vi "输入数据解析.vi"(0 "单个参数补充":dbl, 1 "从板号":dbl=1.0, 2 "主板二维码":string="BNET01", 3 "从板二维码":string="BNET01", 5 "主板引用":refnum<vi>, 7 "从板引用":refnum<vi>, 9 "主板选项":string="三级故障阀值", 11 "枚举":enum16{"主板", "从板"}(ring), 12 "快换":bool caption="快换写入") -> (4 "输出数组":dbl[][](array[numeric]), 6 "数组长度":dbl[](array[numeric]), 8 "循环次数":i32, 10 "命令":u32, 14 "名称":string[](array[string]), 15 "命令序号":u32[](array[numeric]))   [LabVIEW 2013] (continued)
            n304 = Insert Into Array(array=w672, new element=w674) -> (w673:dbl[])  [unwired: 1 in]
          }
          n305 = Build Array(62.0 ("元素")) -> (w664:dbl[])
          n306 = Insert Into Array(array=w650, index=w648, new element #1=w648, new element #2=w648) -> (w649:dbl[])
          n307 = Build Array(u32 5 ("命令序号")) -> (w662:u32[])
          n308 = Build Array(w649) -> (w657:dbl[][])
          n309 = Build Array("温度个数") -> (w653:string[])
        }
        frame "温度起始值" {
          n310 = Unbundle By Name(w702) -> ("项目信息"=w697:refnum<vi>)
          n311 = property class="Tbl (严格)"(reference=w697) -> ("Value"=w696:string[][])  [unwired: 1 in, 2 out]
          n312 = Index Array(array=w696, index (col)=1 ("禁用的索引 (列)")) -> (element=w698:string[])  [unwired: 1 in]
          n313 = Increment(x=w689) -> (x+1=w691:dbl)
          n314 = Multiply(x=w689, y=3.0) -> (x*y=w687:dbl)
          n315 = Add(x=w687, y=23.0) -> (x+y=w690:dbl)
          n316 = Array Subset(array=w698, index=w690, length=w691) -> (w700:string[])
          n317 = Fract/Exp String To Number(string=w700) -> (number=w685:dbl[])  [unwired: 4 out]
          n318 = for {
            tunnel: w685 -> [w709] mode=indexing
            shift-right: [w704] -> w684
            shift-left: dbl[] [] -> [w703]
            n319 = Quotient & Remainder(x=w709, y=256.0) -> (x-y*floor(x/y)=w706:dbl, floor(x/y)=w707:dbl)
            n320 = Build Array(w707, w706) -> (w705:dbl[])
            n321 = Insert Into Array(array=w703, new element=w705) -> (w704:dbl[])  [unwired: 1 in]
          }
          n322 = Build Array(62.0 ("元素")) -> (w695:dbl[])
          n323 = Build Array(u32 6 ("命令序号")) -> (w693:u32[])
          n324 = Build Array(w684) -> (w683:dbl[][])
          n325 = Build Array("温度起始值") -> (w679:string[])
        }
        frame "SOC" {
          # "SOC"
          n326 = Unbundle By Name(w730) -> ("一级故障 4"=w725:refnum<vi>)
          n327 = property class="Clust (严格)"(reference=w725) -> ("Value"=w724:T3)  [unwired: 1 in, 2 out]
          n328 = Unbundle By Name(w724) -> ("SOC(%)"=w722:dbl)
          n329 = call "输入分辨率计算-EV05.vi"("1字节?"=FALSE, "数值"=w722, "分辨率"=0.1) -> ("低字节"=w719:dbl, "高字节1"=w720:dbl)  [unwired: 2 in, 5 out]
          n330 = Build Array(w720, w719) -> (w731:dbl[])
          n331 = Two Button Dialog(message="输入SOC前请确认实际容量己输入" ("消息"), 1:"取消" ("F按钮名称（“取消”）"), 2:"确定" ("T按钮名称（“确定”）")) -> (T button?=w713:bool)
          n332 = case shown="假" w713 {
            tunnel: [0 1] -> w726
            frame False {
            }
            frame True {
            }
          }
          n333 = Build Array("SOC") -> (w714:string[])
          n334 = Build Array(w731) -> (w718:dbl[][])
          n335 = Build Array(2.0 ("单个参数补充")) -> (w717:dbl[])
          n336 = Build Array(u32 7 ("命令序号")) -> (w716:u32[])
        }
        frame "电池额定实际容量" {
          w747 = 256.0 ("y")
          w756 = 256.0 ("y")
          # "电池额定容量,实际容量"
          n337 = Unbundle By Name(w767) -> ("一级故障 4"=w754:refnum<vi>)
          n338 = property class="Clust (严格)"(reference=w754) -> ("Value"=w753:T3)  [unwired: 1 in, 2 out]
          n339 = Unbundle By Name(w753) -> ("电池额定容量(A)"=w751:dbl, "电池实际容量(A)"=w750:dbl)
          n340 = call "输入分辨率计算-EV05.vi"("1字节?"=TRUE, "数值 2"=w750, "数值"=w751, "分辨率"=0.001) -> ("高字节 2"=w743:dbl, "高字节1"=w749:dbl)  [unwired: 1 in, 5 out]
          n341 = Quotient & Remainder(x=w749, y=w756) -> (x-y*floor(x/y)=w760:dbl, floor(x/y)=w762:dbl)
          n342 = Quotient & Remainder(x=w743, y=w747) -> (x-y*floor(x/y)=w739:dbl, floor(x/y)=w744:dbl)
          n343 = Quotient & Remainder(x=w762, y=w756) -> (x-y*floor(x/y)=w759:dbl, floor(x/y)=w761:dbl)
          n344 = Quotient & Remainder(x=w744, y=w747) -> (x-y*floor(x/y)=w740:dbl, floor(x/y)=w745:dbl)
          n345 = Quotient & Remainder(x=w761, y=w756) -> (x-y*floor(x/y)=w758:dbl, floor(x/y)=w757:dbl)
          n346 = Quotient & Remainder(x=w745, y=w747) -> (x-y*floor(x/y)=w741:dbl, floor(x/y)=w746:dbl)
          n347 = Quotient & Remainder(x=w746, y=w747) -> (x-y*floor(x/y)=w742:dbl)  [unwired: 1 out]
          n348 = Quotient & Remainder(x=w757, y=w756) -> (x-y*floor(x/y)=w755:dbl)  [unwired: 1 out]
          n349 = Build Array(w755, w758, w759, w760, w742, w741, w740, w739) -> (w768:dbl[])
          n350 = Build Array(w768) -> (w738:dbl[][])
          n351 = Build Array(8.0 ("单个参数补充")) -> (w737:dbl[])
          n352 = Build Array(u32 8 ("命令序号")) -> (w736:u32[])
          n353 = Build Array("电池额定实际容量") -> (w734:string[])
        }
        frame "配置文件版本" {
          w780 = 8 ("长度")
          # "配置文件版本"
          n354 = Unbundle By Name(w782) -> ("一级故障 4"=w776:refnum<vi>)
          n355 = property class="Clust (严格)"(reference=w776) -> ("Value"=w775:T3)  [unwired: 1 in, 2 out]
          n356 = Unbundle By Name(w775) -> ("配置文件版本"=w774:string)
          n357 = String To Byte Array(string=w774) -> (unsigned byte array=w777:u8[])
          n358 = Array Subset(array=w777, length=w780) -> (w783:u8[])  [unwired: 1 in]
          n359 = Build Array(w783) -> (w773:u8[][])
          n360 = Build Array(w780) -> (w772:i32[])
          n361 = Build Array(u32 9 ("命令序号")) -> (w771:u32[])
          n362 = Build Array("配置文件版本") -> (w769:string[])
        }
        frame "参数修改记录" {
          n363 = Unbundle By Name(w806) -> ("一级故障 4"=w795:refnum<vi>)
          n364 = property class="Clust (严格)"(reference=w795) -> ("Value"=w794:T3)  [unwired: 1 in, 2 out]
          n365 = Unbundle By Name(w794) -> ("使用者"=w793:dbl)
          n366 = Quotient & Remainder(x=w793, y=256.0) -> (x-y*floor(x/y)=w790:dbl, floor(x/y)=w791:dbl)
          n367 = call "当前时间解析-8.6.vi"("需要秒？(T)"=TRUE) -> ("年"=w801:u8, "月"=w800:u8, "日"=w799:u8, "时"=w798:u8, "分"=w797:u8, "秒"=w796:u8)  [unwired: 13 out]
          n368 = Build Array(w791, w790, w801, w800, w799, w798, w797, w796) -> (w807:dbl[])
          n369 = Build Array(w807) -> (w789:dbl[][])
          n370 = Build Array(8.0 ("单个参数补充")) -> (w788:dbl[])
          n371 = Build Array(u32 10 ("命令序号")) -> (w787:u32[])
          n372 = Build Array("参数修改记录") -> (w784:string[])
        }
        frame "校正时钟" {
          n373 = call "当前时间解析-8.6.vi"("需要秒？(T)"=TRUE) -> ("年"=w819:u8, "月"=w818:u8, "日"=w817:u8, "时"=w816:u8, "分"=w815:u8, "秒"=w814:u8)  [unwired: 13 out]
          n374 = Build Array(w819, w818, w817, w816, w815, w814) -> (w824:u8[])
          n375 = Build Array(w824) -> (w813:u8[][])
          n376 = Build Array(6.0 ("单个参数补充")) -> (w812:dbl[])
          n377 = Build Array(u32 14 ("命令序号")) -> (w811:u32[])
          n378 = Build Array("校正时钟") -> (w808:string[])
        }
        frame "车牌号" {
          w836 = 8 ("长度")
          # "车牌号"
          n379 = Unbundle By Name(w838) -> ("一级故障 4"=w832:refnum<vi>)
          n380 = property class="Clust (严格)"(reference=w832) -> ("Value"=w831:T3)  [unwired: 1 in, 2 out]
          n381 = Unbundle By Name(w831) -> ("车架(牌)号"=w830:string)
          n382 = String To Byte Array(string=w830) -> (unsigned byte array=w833:u8[])
          n383 = Array Subset(array=w833, length=w836) -> (w839:u8[])  [unwired: 1 in]
          n384 = Build Array(w839) -> (w829:u8[][])
          n385 = Build Array(w836) -> (w828:i32[])
          n386 = Build Array("车牌号") -> (w825:string[])
          n387 = Build Array(u32 11 ("命令序号")) -> (w827:u32[])
        }
        frame "SOH" {
          n388 = Unbundle By Name(w856) -> ("一级故障 4"=w851:refnum<vi>)
          n389 = property class="Clust (严格)"(reference=w851) -> ("Value"=w850:T3)  [unwired: 1 in, 2 out]
          n390 = Unbundle By Name(w850) -> ("SOH(%)"=w849:dbl)
          n391 = call "输入分辨率计算-EV05.vi"("1字节?"=FALSE, "数值"=w849, "分辨率"=0.1) -> ("低字节"=w845:dbl, "高字节1"=w846:dbl)  [unwired: 2 in, 5 out]
          n392 = Build Array(w846, w845) -> (w857:dbl[])
          n393 = Build Array(w857) -> (w844:dbl[][])
          n394 = Build Array(2.0 ("单个参数补充")) -> (w843:dbl[])
          n395 = Build Array("SOH") -> (w840:string[])
          n396 = Build Array(u32 12 ("命令序号")) -> (w842:u32[])
        }
        frame "一级故障阀值" {
          n397 = Unbundle By Name(w863) -> ("一级故障"=w864:refnum<vi>)
          n398 = property class="Clust (严格)"(reference=w864) -> ("Value"=w862:T4)  [unwired: 1 in, 2 out]
          n399 = for {
            N: 17 -> [_]
            tunnel: w862 -> [w874]
            shift-right: [w871] -> w868
            shift-left: dbl[] [] -> [w872]
            i -> [w875]
            n400 = case shown="11" w875 {
              tunnel: w874 -> [w877 w884 w891 w898 w905 w911 w919 w927 w935 w943 w951 w959 w967 w975 w985 w992 w996]
              tunnel: [w878 w885 w893 w900 w906 w914 w922 w930 w938 w946 w954 w960 w969 w977 w984 w991 w998] -> w873
              frame 0, Default {
                # "总电压过高"
                n401 = Unbundle By Name(w877) -> ("总电压过高"=w876:dbl)
                n402 = call "输入分辨率计算-EV05.vi"("1字节?"=FALSE, "数值"=w876, "分辨率"=0.1) -> ("低字节"=w880:dbl, "高字节1"=w879:dbl)  [unwired: 2 in, 5 out]
                n403 = Build Array(w879, w880) -> (w878:dbl[])
              }
              frame 1 {
                # "总电压过低"
                n404 = Unbundle By Name(w884) -> ("总电压过低"=w883:dbl)
                n405 = call "输入分辨率计算-EV05.vi"("1字节?"=FALSE, "数值"=w883, "分辨率"=0.1) -> ("低字节"=w887:dbl, "高字节1"=w886:dbl)  [unwired: 2 in, 5 out]
                n406 = Build Array(w886, w887) -> (w885:dbl[])
              }
              frame 2 {
                # "温度过高"
                n407 = Unbundle By Name(w891) -> ("温度过高"=w890:dbl)
                n408 = call "输入分辨率计算-EV05.vi"("1字节?"=TRUE, "数值"=w890, "偏移量"=-40.0, "分辨率"=1.0) -> ("高字节1"=w894:dbl)  [unwired: 1 in, 6 out]
                n409 = Build Array(w894) -> (w893:dbl[])
              }
              frame 3 {
                # "温度过低"
                n410 = Unbundle By Name(w898) -> ("温度过低"=w897:dbl)
                n411 = call "输入分辨率计算-EV05.vi"("1字节?"=TRUE, "数值"=w897, "偏移量"=-40.0, "分辨率"=1.0) -> ("高字节1"=w901:dbl)  [unwired: 1 in, 6 out]
                n412 = Build Array(w901) -> (w900:dbl[])
              }
              frame 4 {
                # "整组温度不均衡"
                n413 = Unbundle By Name(w905) -> ("整组温度不均衡"=w904:dbl)
                n414 = call "输入分辨率计算-EV05.vi"("1字节?"=TRUE, "数值"=w904, "分辨率"=1.0) -> ("高字节1"=w907:dbl)  [unwired: 2 in, 6 out]
                n415 = Build Array(w907) -> (w906:dbl[])
              }
              frame 5 {
                # "单组电压不均衡"
                n416 = Unbundle By Name(w911) -> ("单组电压不均衡"=w910:dbl)
                n417 = call "输入分辨率计算-EV05.vi"("1字节?"=FALSE, "数值"=w910, "偏移量"=0.0, "分辨率"=0.001) -> ("低字节"=w912:dbl, "高字节1"=w915:dbl)  [unwired: 1 in, 5 out]
                n418 = Build Array(w915, w912) -> (w914:dbl[])
              }
              frame 6 {
                # "整组电压不均衡"
                n419 = Unbundle By Name(w919) -> ("整组电压不均衡"=w918:dbl)
                n420 = call "输入分辨率计算-EV05.vi"("1字节?"=FALSE, "数值"=w918, "偏移量"=0.0, "分辨率"=0.001) -> ("低字节"=w920:dbl, "高字节1"=w923:dbl)  [unwired: 1 in, 5 out]
                n421 = Build Array(w923, w920) -> (w922:dbl[])
              }
              frame 7 {
                # "单体电压过高"
                n422 = Unbundle By Name(w927) -> ("单体电压过高"=w926:dbl)
                n423 = call "输入分辨率计算-EV05.vi"("1字节?"=FALSE, "数值"=w926, "偏移量"=0.0, "分辨率"=0.001) -> ("低字节"=w928:dbl, "高字节1"=w931:dbl)  [unwired: 1 in, 5 out]
                n424 = Build Array(w931, w928) -> (w930:dbl[])
              }
              frame 8 {
                # "单体电压过低"
                n425 = Unbundle By Name(w935) -> ("单体电压过低"=w934:dbl)
                n426 = call "输入分辨率计算-EV05.vi"("1字节?"=FALSE, "数值"=w934, "偏移量"=0.0, "分辨率"=0.001) -> ("低字节"=w936:dbl, "高字节1"=w939:dbl)  [unwired: 1 in, 5 out]
                n427 = Build Array(w939, w936) -> (w938:dbl[])
              }
              frame 9 {
                # "充电电流过高"
                n428 = Unbundle By Name(w943) -> ("充电电流过高"=w942:dbl)
                n429 = call "输入分辨率计算-EV05.vi"("1字节?"=FALSE, "数值"=w942, "偏移量"=0.0, "分辨率"=0.1) -> ("低字节"=w944:dbl, "高字节1"=w947:dbl)  [unwired: 1 in, 5 out]
                n430 = Build Array(w947, w944) -> (w946:dbl[])
              }
              frame 10 {
                # "放电电流过高"
                n431 = Unbundle By Name(w951) -> ("放电电流过高"=w950:dbl)
                n432 = call "输入分辨率计算-EV05.vi"("1字节?"=FALSE, "数值"=w950, "偏移量"=0.0, "分辨率"=0.1) -> ("低字节"=w952:dbl, "高字节1"=w955:dbl)  [unwired: 1 in, 5 out]
                n433 = Build Array(w955, w952) -> (w954:dbl[])
              }
              frame 11 {
                # "单组温度不均衡"
                n434 = Unbundle By Name(w959) -> ("单组温度不均衡"=w958:dbl)
                n435 = call "输入分辨率计算-EV05.vi"("1字节?"=TRUE, "数值"=w958, "分辨率"=1.0) -> ("高字节1"=w961:dbl)  [unwired: 2 in, 6 out]
                n436 = Build Array(w961) -> (w960:dbl[])
              }
              frame 12 {
                # "SOC过高"
                n437 = Unbundle By Name(w967) -> ("SOC过高"=w966:dbl)
                n438 = call "输入分辨率计算-EV05.vi"("1字节?"=FALSE, "数值"=w966, "偏移量"=0.0, "分辨率"=0.1) -> ("低字节"=w964:dbl, "高字节1"=w965:dbl)  [unwired: 1 in, 5 out]
                n439 = Build Array(w965, w964) -> (w969:dbl[])
              }
              frame 13 {
                # "SOC过低"
                n440 = Unbundle By Name(w975) -> ("SOC过低"=w974:dbl)
                n441 = call "输入分辨率计算-EV05.vi"("1字节?"=FALSE, "数值"=w974, "偏移量"=0.0, "分辨率"=0.1) -> ("低字节"=w972:dbl, "高字节1"=w973:dbl)  [unwired: 1 in, 5 out]
                n442 = Build Array(w973, w972) -> (w977:dbl[])
              }
              frame 14 {
                # "内阻过大"
                n443 = Unbundle By Name(w985) -> ("内阻过大"=w983:dbl)
                n444 = call "输入分辨率计算-EV05.vi"("1字节?"=TRUE, "数值"=w983, "分辨率"=0.1) -> ("高字节1"=w980:dbl)  [unwired: 2 in, 6 out]
                n445 = Build Array(w980) -> (w984:dbl[])
              }
              frame 15 {
                # "极柱温度过高"
                n446 = Unbundle By Name(w992) -> ("极柱温度过高"=w990:dbl)
                n447 = call "输入分辨率计算-EV05.vi"("1字节?"=TRUE, "数值"=w990, "偏移量"=-40.0, "分辨率"=1.0) -> ("高字节1"=w987:dbl)  [unwired: 1 in, 6 out]
                n448 = Build Array(w987) -> (w991:dbl[])
              }
              frame 16 {
                # "SOH过低"
                n449 = Unbundle By Name(w996) -> ("SOH过低"=w995:dbl)
                n450 = call "输入分辨率计算-EV05.vi"("1字节?"=FALSE, "数值"=w995, "偏移量"=0.0, "分辨率"=0.1) -> ("低字节"=w994:dbl, "高字节1"=w993:dbl)  [unwired: 1 in, 5 out]
                n451 = Build Array(w993, w994) -> (w998:dbl[])
              }
            }
            n452 = Insert Into Array(array=w872, new element=w873) -> (w871:dbl[])  [unwired: 1 in]
          }
          n453 = Build Array(w868) -> (w867:dbl[][])
          n454 = Build Array("一级故障阀值") -> (w858:string[])
        }
        frame "温度过高" {
          n455 = Unbundle By Name(w1006) -> ("一级故障"=w1007:refnum<vi>)
          n456 = property class="Clust (严格)"(reference=w1007) -> ("Value"=w1005:T4)  [unwired: 1 in, 2 out]
          n457 = for {
            N: 17 -> [_]
            tunnel: w1005 -> [w1017]
            shift-right: [w1014] -> w1011
            shift-left: dbl[] [] -> [w1015]
            i -> [w1018]
            n458 = case shown="13" w1018 {
              tunnel: w1017 -> [w1019 w1030 w1041 w1051 w1061 w1071 w1083 w1095 w1107 w1119 w1131 w1143 w1157 w1179 w1191 w1200 w1209]
              tunnel: [w1020 w1031 w1042 w1052 w1062 w1073 w1085 w1097 w1109 w1121 w1133 w1144 w1166 w1182 w1190 w1199 w1211] -> w1016
              frame 0, Default {
                # "总电压过高"
                n459 = disable-structure shown="启用" {
                  disable-tunnel: [w1026 w1029] -> w1022
                  disable-tunnel: [w1025 w1029] -> w1021
                  disable-tunnel: w1019 -> [w1024 _]
                  frame Disabled {
                    n460 = Unbundle By Name(w1024) -> ("总电压过高"=w1023:dbl)
                    n461 = call "输入分辨率计算-EV05.vi"("1字节?"=FALSE, "数值"=w1023, "分辨率"=0.1) -> ("低字节"=w1026:dbl, "高字节1"=w1025:dbl)  [unwired: 2 in, 5 out]
                  }
                  frame Enabled {
                    w1029 = 255 ("高字节1")
                  }
                }
                n462 = Build Array(w1021, w1022) -> (w1020:i32[])
              }
              frame 1 {
                # "总电压过低"
                n463 = disable-structure shown="启用" {
                  disable-tunnel: [w1037 w1040] -> w1033
                  disable-tunnel: [w1036 w1040] -> w1032
                  disable-tunnel: w1030 -> [w1035 _]
                  frame Disabled {
                    n464 = Unbundle By Name(w1035) -> ("总电压过低"=w1034:dbl)
                    n465 = call "输入分辨率计算-EV05.vi"("1字节?"=FALSE, "数值"=w1034, "分辨率"=0.1) -> ("低字节"=w1037:dbl, "高字节1"=w1036:dbl)  [unwired: 2 in, 5 out]
                  }
                  frame Enabled {
                    w1040 = 255 ("高字节1")
                  }
                }
                n466 = Build Array(w1032, w1033) -> (w1031:i32[])
              }
              frame 2 {
                # "温度过高"
                n467 = disable-structure shown="启用" {
                  disable-tunnel: [w1047 255 ("高字节1")] -> w1043
                  disable-tunnel: w1041 -> [w1045 _]
                  frame Enabled {
                    n468 = Unbundle By Name(w1045) -> ("温度过高"=w1044:dbl)
                    n469 = call "输入分辨率计算-EV05.vi"("1字节?"=TRUE, "数值"=w1044, "偏移量"=-40.0, "分辨率"=1.0) -> ("高字节1"=w1047:dbl)  [unwired: 1 in, 6 out]
                  }
                  frame Disabled {
                  }
                }
                n470 = Build Array(w1043) -> (w1042:dbl[])
              }
              frame 3 {
                # "温度过低"
                n471 = disable-structure shown="启用" {
                  disable-tunnel: [w1057 255 ("高字节1")] -> w1053
                  disable-tunnel: w1051 -> [w1055 _]
                  frame Disabled {
                    n472 = Unbundle By Name(w1055) -> ("温度过低"=w1054:dbl)
                    n473 = call "输入分辨率计算-EV05.vi"("1字节?"=TRUE, "数值"=w1054, "偏移量"=-40.0, "分辨率"=1.0) -> ("高字节1"=w1057:dbl)  [unwired: 1 in, 6 out]
                  }
                  frame Enabled {
                  }
                }
                n474 = Build Array(w1053) -> (w1052:i32[])
              }
              frame 4 {
                # "整组温度不均衡"
                n475 = disable-structure shown="启用" {
                  disable-tunnel: [w1067 255 ("高字节1")] -> w1063
                  disable-tunnel: w1061 -> [w1065 _]
                  frame Disabled {
                    n476 = Unbundle By Name(w1065) -> ("整组温度不均衡"=w1064:dbl)
                    n477 = call "输入分辨率计算-EV05.vi"("1字节?"=TRUE, "数值"=w1064, "偏移量"=0.0, "分辨率"=1.0) -> ("高字节1"=w1067:dbl)  [unwired: 1 in, 6 out]
                  }
                  frame Enabled {
                  }
                }
                n478 = Build Array(w1063) -> (w1062:i32[])
              }
              frame 5 {
                # "单组电压不均衡"
                n479 = disable-structure shown="启用" {
                  disable-tunnel: [w1079 w1082] -> w1074
                  disable-tunnel: [w1077 w1082] -> w1072
                  disable-tunnel: w1071 -> [w1076 _]
                  frame Disabled {
                    n480 = Unbundle By Name(w1076) -> ("单组电压不均衡"=w1075:dbl)
                    n481 = call "输入分辨率计算-EV05.vi"("1字节?"=FALSE, "数值"=w1075, "偏移量"=0.0, "分辨率"=0.001) -> ("低字节"=w1077:dbl, "高字节1"=w1079:dbl)  [unwired: 1 in, 5 out]
                  }
                  frame Enabled {
                    w1082 = 255 ("高字节1")
                  }
                }
                n482 = Build Array(w1074, w1072) -> (w1073:i32[])
              }
              frame 6 {
                # "整组电压不均衡"
                n483 = disable-structure shown="启用" {
                  disable-tunnel: [w1091 w1094] -> w1086
                  disable-tunnel: [w1089 w1094] -> w1084
                  disable-tunnel: w1083 -> [w1088 _]
                  frame Disabled {
                    n484 = Unbundle By Name(w1088) -> ("整组电压不均衡"=w1087:dbl)
                    n485 = call "输入分辨率计算-EV05.vi"("1字节?"=FALSE, "数值"=w1087, "偏移量"=0.0, "分辨率"=0.001) -> ("低字节"=w1089:dbl, "高字节1"=w1091:dbl)  [unwired: 1 in, 5 out]
                  }
                  frame Enabled {
                    w1094 = 255 ("高字节1")
                  }
                }
                n486 = Build Array(w1086, w1084) -> (w1085:i32[])
              }
              frame 7 {
                # "单体电压过高"
                n487 = disable-structure shown="启用" {
                  disable-tunnel: [w1103 w1106] -> w1098
                  disable-tunnel: [w1101 w1106] -> w1096
                  disable-tunnel: w1095 -> [w1100 _]
                  frame Disabled {
                    n488 = Unbundle By Name(w1100) -> ("单体电压过高"=w1099:dbl)
                    n489 = call "输入分辨率计算-EV05.vi"("1字节?"=FALSE, "数值"=w1099, "偏移量"=0.0, "分辨率"=0.001) -> ("低字节"=w1101:dbl, "高字节1"=w1103:dbl)  [unwired: 1 in, 5 out]
                  }
                  frame Enabled {
                    w1106 = 255 ("高字节1")
                  }
                }
                n490 = Build Array(w1098, w1096) -> (w1097:i32[])
              }
              frame 8 {
                # "单体电压过低"
                n491 = disable-structure shown="启用" {
                  disable-tunnel: [w1115 w1118] -> w1110
                  disable-tunnel: [w1113 w1118] -> w1108
                  disable-tunnel: w1107 -> [w1112 _]
                  frame Disabled {
                    n492 = Unbundle By Name(w1112) -> ("单体电压过低"=w1111:dbl)
                    n493 = call "输入分辨率计算-EV05.vi"("1字节?"=FALSE, "数值"=w1111, "偏移量"=0.0, "分辨率"=0.001) -> ("低字节"=w1113:dbl, "高字节1"=w1115:dbl)  [unwired: 1 in, 5 out]
                  }
                  frame Enabled {
                    w1118 = 255 ("高字节1")
                  }
                }
                n494 = Build Array(w1110, w1108) -> (w1109:i32[])
              }
              frame 9 {
                # "充电电流过高"
                n495 = disable-structure shown="启用" {
                  disable-tunnel: [w1127 w1130] -> w1122
                  disable-tunnel: [w1125 w1130] -> w1120
                  disable-tunnel: w1119 -> [w1124 _]
                  frame Disabled {
                    n496 = Unbundle By Name(w1124) -> ("充电电流过高"=w1123:dbl)
                    n497 = call "输入分辨率计算-EV05.vi"("1字节?"=FALSE, "数值"=w1123, "偏移量"=-3000.0, "分辨率"=0.1) -> ("低字节"=w1125:dbl, "高字节1"=w1127:dbl)  [unwired: 1 in, 5 out]
                  }
                  frame Enabled {
                    w1130 = 255 ("高字节1")
                  }
                }
                n498 = Build Array(w1122, w1120) -> (w1121:i32[])
              }
              frame 10 {
                # "放电电流过高"
                n499 = disable-structure shown="启用" {
                  disable-tunnel: [w1139 w1142] -> w1134
                  disable-tunnel: [w1137 w1142] -> w1132
                  disable-tunnel: w1131 -> [w1136 _]
                  frame Disabled {
                    n500 = Unbundle By Name(w1136) -> ("放电电流过高"=w1135:dbl)
                    n501 = call "输入分辨率计算-EV05.vi"("1字节?"=FALSE, "数值"=w1135, "偏移量"=-3000.0, "分辨率"=0.1) -> ("低字节"=w1137:dbl, "高字节1"=w1139:dbl)  [unwired: 1 in, 5 out]
                  }
                  frame Enabled {
                    w1142 = 255 ("高字节1")
                  }
                }
                n502 = Build Array(w1134, w1132) -> (w1133:i32[])
              }
              frame 11 {
                # "单组温度不均衡"
                n503 = disable-structure shown="启用" {
                  disable-tunnel: [w1149 255 ("高字节1")] -> w1145
                  disable-tunnel: w1143 -> [w1147 _]
                  frame Disabled {
                    n504 = Unbundle By Name(w1147) -> ("单组温度不均衡"=w1146:dbl)
                    n505 = call "输入分辨率计算-EV05.vi"("1字节?"=TRUE, "数值"=w1146, "偏移量"=0.0, "分辨率"=1.0) -> ("高字节1"=w1149:dbl)  [unwired: 1 in, 6 out]
                  }
                  frame Enabled {
                  }
                }
                n506 = Build Array(w1145) -> (w1144:i32[])
              }
              frame 12 {
                # "SOC过高"
                n507 = Unbundle By Name(w1157) -> ("SOC过高"=w1156:dbl)
                n508 = call "输入分辨率计算-EV05.vi"("1字节?"=FALSE, "数值"=w1156, "偏移量"=0.0, "分辨率"=0.1) -> ("低字节"=w1158:dbl, "高字节1"=w1159:dbl)  [unwired: 1 in, 5 out]
                n509 = call "二进制解析-8.6.vi"("索引"=4, "数值"=w1159) -> ("低位子数组"=w1162:i32[])  [unwired: 3 out]
                n510 = call "二进制解析-8.6.vi"("索引"=4, "数值"=w1158) -> ("低位子数组"=w1154:i32[], "高位子数组"=w1161:i32[])  [unwired: 2 out]
                n511 = Insert Into Array(array=w1162, new element=w1161) -> (w1160:i32[])  [unwired: 1 in]
                n512 = call "数值二进制转十进制-8.6.vi"("子数组"=w1160) -> ("十进制数值"=w1155:i32)  [unwired: 4 out]
                n513 = disable-structure shown="启用" {
                  disable-tunnel: w1155 -> [w1170 _]
                  disable-tunnel: [w1170 255 ("高字节1")] -> w1153
                  disable-tunnel: [w1169 i32[] [] ("低位子数组 20")] -> _
                  disable-tunnel: w1154 -> [w1169 _]
                  frame Disabled {
                  }
                  frame Enabled {
                  }
                }
                n514 = Build Array(w1153, w1153) -> (w1166:i32[])
              }
              frame 13 {
                # "SOC过低"
                n515 = Unbundle By Name(w1179) -> ("SOC过低"=w1178:dbl)
                n516 = call "输入分辨率计算-EV05.vi"("1字节?"=FALSE, "数值"=w1178, "偏移量"=0.0, "分辨率"=0.1) -> ("低字节"=w1176:dbl, "高字节1"=w1177:dbl)  [unwired: 1 in, 5 out]
                n517 = call "二进制解析-8.6.vi"("索引"=4, "数值"=w1177) -> ("低位子数组"=w1174:i32[])  [unwired: 3 out]
                n518 = disable-structure shown="启用" {
                  disable-tunnel: w1176 -> [w1186 _]
                  disable-tunnel: [w1186 255 ("高字节1")] -> w1175
                  disable-tunnel: w1174 -> [w1185 _]
                  disable-tunnel: [_ 255 ("高字节1")] -> w1173
                  frame Disabled {
                    (unwired) i32[] [] ("低位子数组 4")
                  }
                  frame Enabled {
                  }
                }
                n519 = Build Array(w1173, w1175) -> (w1182:i32[])
              }
              frame 14 {
                # "内阻过大"
                n520 = disable-structure shown="启用" {
                  disable-tunnel: w1191 -> [w1196 _]
                  disable-tunnel: [w1192 255 ("高字节1")] -> w1189
                  frame Disabled {
                    n521 = Unbundle By Name(w1196) -> ("内阻过大"=w1195:dbl)
                    n522 = call "输入分辨率计算-EV05.vi"("1字节?"=TRUE, "数值"=w1195, "分辨率"=0.1) -> ("高字节1"=w1192:dbl)  [unwired: 2 in, 6 out]
                  }
                  frame Enabled {
                  }
                }
                n523 = Build Array(w1189) -> (w1190:i32[])
              }
              frame 15 {
                # "极柱温度过高"
                n524 = disable-structure shown="启用" {
                  disable-tunnel: w1200 -> [w1206 _]
                  disable-tunnel: [w1202 255 ("高字节1")] -> w1198
                  frame Disabled {
                    n525 = Unbundle By Name(w1206) -> ("极柱温度过高"=w1205:dbl)
                    n526 = call "输入分辨率计算-EV05.vi"("1字节?"=TRUE, "数值"=w1205, "偏移量"=-40.0, "分辨率"=1.0) -> ("高字节1"=w1202:dbl)  [unwired: 1 in, 6 out]
                  }
                  frame Enabled {
                  }
                }
                n527 = Build Array(w1198) -> (w1199:i32[])
              }
              frame 16 {
                # "SOH过低"
                n528 = disable-structure shown="启用" {
                  disable-tunnel: [w1223 w1231] -> w1210
                  disable-tunnel: w1209 -> [w1220 _]
                  disable-tunnel: [w1212 w1231] -> w1208
                  frame Disabled {
                    n529 = Unbundle By Name(w1220) -> ("SOH过低"=w1219:dbl)
                    n530 = call "输入分辨率计算-EV05.vi"("1字节?"=FALSE, "数值"=w1219, "偏移量"=0.0, "分辨率"=0.1) -> ("低字节"=w1221:dbl, "高字节1"=w1222:dbl)  [unwired: 1 in, 5 out]
                    n531 = call "二进制解析-8.6.vi"("索引"=4, "数值"=w1222) -> ("低位子数组"=w1225:i32[])  [unwired: 3 out]
                    n532 = call "二进制解析-8.6.vi"("索引"=4, "数值"=w1221) -> ("低位子数组"=w1214:i32[], "高位子数组"=w1224:i32[])  [unwired: 2 out]
                    n533 = call "二进制解析-8.6.vi"("索引"=4, "数值"=0) -> ("低位子数组"=w1215:i32[])  [unwired: 3 out]
                    n534 = Insert Into Array(array=w1225, new element=w1224) -> (w1218:i32[])  [unwired: 1 in]
                    n535 = Insert Into Array(array=w1214, new element=w1215) -> (w1213:i32[])  [unwired: 1 in]
                    n536 = call "数值二进制转十进制-8.6.vi"("子数组"=w1218) -> ("十进制数值"=w1223:i32)  [unwired: 4 out]
                    n537 = call "数值二进制转十进制-8.6.vi"("子数组"=w1213) -> ("十进制数值"=w1212:i32)  [unwired: 4 out]
                  }
                  frame Enabled {
                    w1231 = 255 ("高字节1")
                  }
                }
                n538 = Build Array(w1210, w1208) -> (w1211:i32[])
              }
            }
            n539 = Insert Into Array(array=w1015, new element=w1016) -> (w1014:dbl[])  [unwired: 1 in]
          }
          n540 = Build Array(w1011) -> (w1010:dbl[][])
          n541 = Build Array("一级故障阀值") -> (w1001:string[])
        }
        frame "总电压过高" {
          n542 = Unbundle By Name(w1237) -> ("一级故障"=w1238:refnum<vi>)
          n543 = property class="Clust (严格)"(reference=w1238) -> ("Value"=w1236:T4)  [unwired: 1 in, 2 out]
          n544 = for {
            N: 17 -> [_]
            tunnel: w1236 -> [w1248]
            shift-right: [w1245] -> w1242
            shift-left: dbl[] [] -> [w1246]
            i -> [w1249]
            n545 = case shown="13" w1249 {
              tunnel: w1248 -> [w1250 w1261 w1272 w1282 w1292 w1302 w1314 w1326 w1338 w1350 w1362 w1374 w1388 w1410 w1422 w1431 w1440]
              tunnel: [w1251 w1262 w1273 w1283 w1293 w1304 w1316 w1328 w1340 w1352 w1364 w1375 w1397 w1413 w1421 w1430 w1442] -> w1247
              frame 0, Default {
                # "总电压过高"
                n546 = disable-structure shown="启用" {
                  disable-tunnel: [w1257 w1260] -> w1253
                  disable-tunnel: [w1256 w1260] -> w1252
                  disable-tunnel: w1250 -> [w1255 _]
                  frame Enabled {
                    n547 = Unbundle By Name(w1255) -> ("总电压过高"=w1254:dbl)
                    n548 = call "输入分辨率计算-EV05.vi"("1字节?"=FALSE, "数值"=w1254, "分辨率"=0.1) -> ("低字节"=w1257:dbl, "高字节1"=w1256:dbl)  [unwired: 2 in, 5 out]
                  }
                  frame Disabled {
                    w1260 = 255 ("高字节1")
                  }
                }
                n549 = Build Array(w1252, w1253) -> (w1251:dbl[])
              }
              frame 1 {
                # "总电压过低"
                n550 = disable-structure shown="启用" {
                  disable-tunnel: [w1268 w1271] -> w1264
                  disable-tunnel: [w1267 w1271] -> w1263
                  disable-tunnel: w1261 -> [w1266 _]
                  frame Disabled {
                    n551 = Unbundle By Name(w1266) -> ("总电压过低"=w1265:dbl)
                    n552 = call "输入分辨率计算-EV05.vi"("1字节?"=FALSE, "数值"=w1265, "分辨率"=0.1) -> ("低字节"=w1268:dbl, "高字节1"=w1267:dbl)  [unwired: 2 in, 5 out]
                  }
                  frame Enabled {
                    w1271 = 255 ("高字节1")
                  }
                }
                n553 = Build Array(w1263, w1264) -> (w1262:i32[])
              }
              frame 2 {
                # "温度过高"
                n554 = disable-structure shown="启用" {
                  disable-tunnel: [w1278 255 ("高字节1")] -> w1274
                  disable-tunnel: w1272 -> [w1276 _]
                  frame Disabled {
                    n555 = Unbundle By Name(w1276) -> ("温度过高"=w1275:dbl)
                    n556 = call "输入分辨率计算-EV05.vi"("1字节?"=TRUE, "数值"=w1275, "偏移量"=-40.0, "分辨率"=1.0) -> ("高字节1"=w1278:dbl)  [unwired: 1 in, 6 out]
                  }
                  frame Enabled {
                  }
                }
                n557 = Build Array(w1274) -> (w1273:i32[])
              }
              frame 3 {
                # "温度过低"
                n558 = disable-structure shown="启用" {
                  disable-tunnel: [w1288 255 ("高字节1")] -> w1284
                  disable-tunnel: w1282 -> [w1286 _]
                  frame Disabled {
                    n559 = Unbundle By Name(w1286) -> ("温度过低"=w1285:dbl)
                    n560 = call "输入分辨率计算-EV05.vi"("1字节?"=TRUE, "数值"=w1285, "偏移量"=-40.0, "分辨率"=1.0) -> ("高字节1"=w1288:dbl)  [unwired: 1 in, 6 out]
                  }
                  frame Enabled {
                  }
                }
                n561 = Build Array(w1284) -> (w1283:i32[])
              }
              frame 4 {
                # "整组温度不均衡"
                n562 = disable-structure shown="启用" {
                  disable-tunnel: [w1298 255 ("高字节1")] -> w1294
                  disable-tunnel: w1292 -> [w1296 _]
                  frame Disabled {
                    n563 = Unbundle By Name(w1296) -> ("整组温度不均衡"=w1295:dbl)
                    n564 = call "输入分辨率计算-EV05.vi"("1字节?"=TRUE, "数值"=w1295, "偏移量"=0.0, "分辨率"=1.0) -> ("高字节1"=w1298:dbl)  [unwired: 1 in, 6 out]
                  }
                  frame Enabled {
                  }
                }
                n565 = Build Array(w1294) -> (w1293:i32[])
              }
              frame 5 {
                # "单组电压不均衡"
                n566 = disable-structure shown="启用" {
                  disable-tunnel: [w1310 w1313] -> w1305
                  disable-tunnel: [w1308 w1313] -> w1303
                  disable-tunnel: w1302 -> [w1307 _]
                  frame Disabled {
                    n567 = Unbundle By Name(w1307) -> ("单组电压不均衡"=w1306:dbl)
                    n568 = call "输入分辨率计算-EV05.vi"("1字节?"=FALSE, "数值"=w1306, "偏移量"=0.0, "分辨率"=0.001) -> ("低字节"=w1308:dbl, "高字节1"=w1310:dbl)  [unwired: 1 in, 5 out]
                  }
                  frame Enabled {
                    w1313 = 255 ("高字节1")
                  }
                }
                n569 = Build Array(w1305, w1303) -> (w1304:i32[])
              }
              frame 6 {
                # "整组电压不均衡"
                n570 = disable-structure shown="启用" {
                  disable-tunnel: [w1322 w1325] -> w1317
                  disable-tunnel: [w1320 w1325] -> w1315
                  disable-tunnel: w1314 -> [w1319 _]
                  frame Disabled {
                    n571 = Unbundle By Name(w1319) -> ("整组电压不均衡"=w1318:dbl)
                    n572 = call "输入分辨率计算-EV05.vi"("1字节?"=FALSE, "数值"=w1318, "偏移量"=0.0, "分辨率"=0.001) -> ("低字节"=w1320:dbl, "高字节1"=w1322:dbl)  [unwired: 1 in, 5 out]
                  }
                  frame Enabled {
                    w1325 = 255 ("高字节1")
                  }
                }
                n573 = Build Array(w1317, w1315) -> (w1316:i32[])
              }
              frame 7 {
                # "单体电压过高"
                n574 = disable-structure shown="启用" {
                  disable-tunnel: [w1334 w1337] -> w1329
                  disable-tunnel: [w1332 w1337] -> w1327
                  disable-tunnel: w1326 -> [w1331 _]
                  frame Disabled {
                    n575 = Unbundle By Name(w1331) -> ("单体电压过高"=w1330:dbl)
                    n576 = call "输入分辨率计算-EV05.vi"("1字节?"=FALSE, "数值"=w1330, "偏移量"=0.0, "分辨率"=0.001) -> ("低字节"=w1332:dbl, "高字节1"=w1334:dbl)  [unwired: 1 in, 5 out]
                  }
                  frame Enabled {
                    w1337 = 255 ("高字节1")
                  }
                }
                n577 = Build Array(w1329, w1327) -> (w1328:i32[])
              }
              frame 8 {
                # "单体电压过低"
                n578 = disable-structure shown="启用" {
                  disable-tunnel: [w1346 w1349] -> w1341
                  disable-tunnel: [w1344 w1349] -> w1339
                  disable-tunnel: w1338 -> [w1343 _]
                  frame Disabled {
                    n579 = Unbundle By Name(w1343) -> ("单体电压过低"=w1342:dbl)
                    n580 = call "输入分辨率计算-EV05.vi"("1字节?"=FALSE, "数值"=w1342, "偏移量"=0.0, "分辨率"=0.001) -> ("低字节"=w1344:dbl, "高字节1"=w1346:dbl)  [unwired: 1 in, 5 out]
                  }
                  frame Enabled {
                    w1349 = 255 ("高字节1")
                  }
                }
                n581 = Build Array(w1341, w1339) -> (w1340:i32[])
              }
              frame 9 {
                # "充电电流过高"
                n582 = disable-structure shown="启用" {
                  disable-tunnel: [w1358 w1361] -> w1353
                  disable-tunnel: [w1356 w1361] -> w1351
                  disable-tunnel: w1350 -> [w1355 _]
                  frame Disabled {
                    n583 = Unbundle By Name(w1355) -> ("充电电流过高"=w1354:dbl)
                    n584 = call "输入分辨率计算-EV05.vi"("1字节?"=FALSE, "数值"=w1354, "偏移量"=-3000.0, "分辨率"=0.1) -> ("低字节"=w1356:dbl, "高字节1"=w1358:dbl)  [unwired: 1 in, 5 out]
                  }
                  frame Enabled {
                    w1361 = 255 ("高字节1")
                  }
                }
                n585 = Build Array(w1353, w1351) -> (w1352:i32[])
              }
              frame 10 {
                # "放电电流过高"
                n586 = disable-structure shown="启用" {
                  disable-tunnel: [w1370 w1373] -> w1365
                  disable-tunnel: [w1368 w1373] -> w1363
                  disable-tunnel: w1362 -> [w1367 _]
                  frame Disabled {
                    n587 = Unbundle By Name(w1367) -> ("放电电流过高"=w1366:dbl)
                    n588 = call "输入分辨率计算-EV05.vi"("1字节?"=FALSE, "数值"=w1366, "偏移量"=-3000.0, "分辨率"=0.1) -> ("低字节"=w1368:dbl, "高字节1"=w1370:dbl)  [unwired: 1 in, 5 out]
                  }
                  frame Enabled {
                    w1373 = 255 ("高字节1")
                  }
                }
                n589 = Build Array(w1365, w1363) -> (w1364:i32[])
              }
              frame 11 {
                # "单组温度不均衡"
                n590 = disable-structure shown="启用" {
                  disable-tunnel: [w1380 255 ("高字节1")] -> w1376
                  disable-tunnel: w1374 -> [w1378 _]
                  frame Disabled {
                    n591 = Unbundle By Name(w1378) -> ("单组温度不均衡"=w1377:dbl)
                    n592 = call "输入分辨率计算-EV05.vi"("1字节?"=TRUE, "数值"=w1377, "偏移量"=0.0, "分辨率"=1.0) -> ("高字节1"=w1380:dbl)  [unwired: 1 in, 6 out]
                  }
                  frame Enabled {
                  }
                }
                n593 = Build Array(w1376) -> (w1375:i32[])
              }
              frame 12 {
                # "SOC过高"
                n594 = Unbundle By Name(w1388) -> ("SOC过高"=w1387:dbl)
                n595 = call "输入分辨率计算-EV05.vi"("1字节?"=FALSE, "数值"=w1387, "偏移量"=0.0, "分辨率"=0.1) -> ("低字节"=w1389:dbl, "高字节1"=w1390:dbl)  [unwired: 1 in, 5 out]
                n596 = call "二进制解析-8.6.vi"("索引"=4, "数值"=w1390) -> ("低位子数组"=w1393:i32[])  [unwired: 3 out]
                n597 = call "二进制解析-8.6.vi"("索引"=4, "数值"=w1389) -> ("低位子数组"=w1385:i32[], "高位子数组"=w1392:i32[])  [unwired: 2 out]
                n598 = Insert Into Array(array=w1393, new element=w1392) -> (w1391:i32[])  [unwired: 1 in]
                n599 = call "数值二进制转十进制-8.6.vi"("子数组"=w1391) -> ("十进制数值"=w1386:i32)  [unwired: 4 out]
                n600 = disable-structure shown="启用" {
                  disable-tunnel: w1386 -> [w1401 _]
                  disable-tunnel: [w1401 255 ("高字节1")] -> w1384
                  disable-tunnel: [w1400 i32[] [] ("低位子数组 20")] -> _
                  disable-tunnel: w1385 -> [w1400 _]
                  frame Disabled {
                  }
                  frame Enabled {
                  }
                }
                n601 = Build Array(w1384, w1384) -> (w1397:i32[])
              }
              frame 13 {
                # "SOC过低"
                n602 = Unbundle By Name(w1410) -> ("SOC过低"=w1409:dbl)
                n603 = call "输入分辨率计算-EV05.vi"("1字节?"=FALSE, "数值"=w1409, "偏移量"=0.0, "分辨率"=0.1) -> ("低字节"=w1407:dbl, "高字节1"=w1408:dbl)  [unwired: 1 in, 5 out]
                n604 = call "二进制解析-8.6.vi"("索引"=4, "数值"=w1408) -> ("低位子数组"=w1405:i32[])  [unwired: 3 out]
                n605 = disable-structure shown="启用" {
                  disable-tunnel: w1407 -> [w1417 _]
                  disable-tunnel: [w1417 255 ("高字节1")] -> w1406
                  disable-tunnel: w1405 -> [w1416 _]
                  disable-tunnel: [_ 255 ("高字节1")] -> w1404
                  frame Disabled {
                    (unwired) i32[] [] ("低位子数组 4")
                  }
                  frame Enabled {
                  }
                }
                n606 = Build Array(w1404, w1406) -> (w1413:i32[])
              }
              frame 14 {
                # "内阻过大"
                n607 = disable-structure shown="启用" {
                  disable-tunnel: w1422 -> [w1427 _]
                  disable-tunnel: [w1423 255 ("高字节1")] -> w1420
                  frame Disabled {
                    n608 = Unbundle By Name(w1427) -> ("内阻过大"=w1426:dbl)
                    n609 = call "输入分辨率计算-EV05.vi"("1字节?"=TRUE, "数值"=w1426, "分辨率"=0.1) -> ("高字节1"=w1423:dbl)  [unwired: 2 in, 6 out]
                  }
                  frame Enabled {
                  }
                }
                n610 = Build Array(w1420) -> (w1421:i32[])
              }
              frame 15 {
                # "极柱温度过高"
                n611 = disable-structure shown="启用" {
                  disable-tunnel: w1431 -> [w1437 _]
                  disable-tunnel: [w1433 255 ("高字节1")] -> w1429
                  frame Disabled {
                    n612 = Unbundle By Name(w1437) -> ("极柱温度过高"=w1436:dbl)
                    n613 = call "输入分辨率计算-EV05.vi"("1字节?"=TRUE, "数值"=w1436, "偏移量"=-40.0, "分辨率"=1.0) -> ("高字节1"=w1433:dbl)  [unwired: 1 in, 6 out]
                  }
                  frame Enabled {
                  }
                }
                n614 = Build Array(w1429) -> (w1430:i32[])
              }
              frame 16 {
                # "SOH过低"
                n615 = disable-structure shown="启用" {
                  disable-tunnel: [w1454 w1462] -> w1441
                  disable-tunnel: w1440 -> [w1451 _]
                  disable-tunnel: [w1443 w1462] -> w1439
                  frame Disabled {
                    n616 = Unbundle By Name(w1451) -> ("SOH过低"=w1450:dbl)
                    n617 = call "输入分辨率计算-EV05.vi"("1字节?"=FALSE, "数值"=w1450, "偏移量"=0.0, "分辨率"=0.1) -> ("低字节"=w1452:dbl, "高字节1"=w1453:dbl)  [unwired: 1 in, 5 out]
                    n618 = call "二进制解析-8.6.vi"("索引"=4, "数值"=w1453) -> ("低位子数组"=w1456:i32[])  [unwired: 3 out]
                    n619 = call "二进制解析-8.6.vi"("索引"=4, "数值"=w1452) -> ("低位子数组"=w1445:i32[], "高位子数组"=w1455:i32[])  [unwired: 2 out]
                    n620 = call "二进制解析-8.6.vi"("索引"=4, "数值"=0) -> ("低位子数组"=w1446:i32[])  [unwired: 3 out]
                    n621 = Insert Into Array(array=w1456, new element=w1455) -> (w1449:i32[])  [unwired: 1 in]
                    n622 = Insert Into Array(array=w1445, new element=w1446) -> (w1444:i32[])  [unwired: 1 in]
                    n623 = call "数值二进制转十进制-8.6.vi"("子数组"=w1449) -> ("十进制数值"=w1454:i32)  [unwired: 4 out]
                    n624 = call "数值二进制转十进制-8.6.vi"("子数组"=w1444) -> ("十进制数值"=w1443:i32)  [unwired: 4 out]
                  }
                  frame Enabled {
                    w1462 = 255 ("高字节1")
                  }
                }
                n625 = Build Array(w1441, w1439) -> (w1442:i32[])
              }
            }
            n626 = Insert Into Array(array=w1246, new element=w1247) -> (w1245:dbl[])  [unwired: 1 in]
          }
          n627 = Build Array(w1242) -> (w1241:dbl[][])
          n628 = Build Array("一级故障阀值") -> (w1232:string[])
        }
        frame "总电压过低" {
          n629 = Unbundle By Name(w1468) -> ("一级故障"=w1469:refnum<vi>)
          n630 = property class="Clust (严格)"(reference=w1469) -> ("Value"=w1467:T4)  [unwired: 1 in, 2 out]
          n631 = for {
            N: 17 -> [_]
            tunnel: w1467 -> [w1479]
            shift-right: [w1476] -> w1473
            shift-left: dbl[] [] -> [w1477]
            i -> [w1480]
            n632 = case shown="13" w1480 {
              tunnel: w1479 -> [w1481 w1492 w1503 w1513 w1523 w1533 w1545 w1557 w1569 w1581 w1593 w1605 w1619 w1641 w1653 w1662 w1671]
              tunnel: [w1482 w1493 w1504 w1514 w1524 w1535 w1547 w1559 w1571 w1583 w1595 w1606 w1628 w1644 w1652 w1661 w1673] -> w1478
              frame 0, Default {
                # "总电压过高"
                n633 = disable-structure shown="启用" {
                  disable-tunnel: [w1488 w1491] -> w1484
                  disable-tunnel: [w1487 w1491] -> w1483
                  disable-tunnel: w1481 -> [w1486 _]
                  frame Disabled {
                    n634 = Unbundle By Name(w1486) -> ("总电压过高"=w1485:dbl)
                    n635 = call "输入分辨率计算-EV05.vi"("1字节?"=FALSE, "数值"=w1485, "分辨率"=0.1) -> ("低字节"=w1488:dbl, "高字节1"=w1487:dbl)  [unwired: 2 in, 5 out]
                  }
                  frame Enabled {
                    w1491 = 255 ("高字节1")
                  }
                }
                n636 = Build Array(w1483, w1484) -> (w1482:i32[])
              }
              frame 1 {
                # "总电压过低"
                n637 = disable-structure shown="启用" {
                  disable-tunnel: [w1499 w1502] -> w1495
                  disable-tunnel: [w1498 w1502] -> w1494
                  disable-tunnel: w1492 -> [w1497 _]
                  frame Enabled {
                    n638 = Unbundle By Name(w1497) -> ("总电压过低"=w1496:dbl)
                    n639 = call "输入分辨率计算-EV05.vi"("1字节?"=FALSE, "数值"=w1496, "分辨率"=0.1) -> ("低字节"=w1499:dbl, "高字节1"=w1498:dbl)  [unwired: 2 in, 5 out]
                  }
                  frame Disabled {
                    w1502 = 255 ("高字节1")
                  }
                }
                n640 = Build Array(w1494, w1495) -> (w1493:dbl[])
              }
              frame 2 {
                # "温度过高"
                n641 = disable-structure shown="启用" {
                  disable-tunnel: [w1509 255 ("高字节1")] -> w1505
                  disable-tunnel: w1503 -> [w1507 _]
                  frame Disabled {
                    n642 = Unbundle By Name(w1507) -> ("温度过高"=w1506:dbl)
                    n643 = call "输入分辨率计算-EV05.vi"("1字节?"=TRUE, "数值"=w1506, "偏移量"=-40.0, "分辨率"=1.0) -> ("高字节1"=w1509:dbl)  [unwired: 1 in, 6 out]
                  }
                  frame Enabled {
                  }
                }
                n644 = Build Array(w1505) -> (w1504:i32[])
              }
              frame 3 {
                # "温度过低"
                n645 = disable-structure shown="启用" {
                  disable-tunnel: [w1519 255 ("高字节1")] -> w1515
                  disable-tunnel: w1513 -> [w1517 _]
                  frame Disabled {
                    n646 = Unbundle By Name(w1517) -> ("温度过低"=w1516:dbl)
                    n647 = call "输入分辨率计算-EV05.vi"("1字节?"=TRUE, "数值"=w1516, "偏移量"=-40.0, "分辨率"=1.0) -> ("高字节1"=w1519:dbl)  [unwired: 1 in, 6 out]
                  }
                  frame Enabled {
                  }
                }
                n648 = Build Array(w1515) -> (w1514:i32[])
              }
              frame 4 {
                # "整组温度不均衡"
                n649 = disable-structure shown="启用" {
                  disable-tunnel: [w1529 255 ("高字节1")] -> w1525
                  disable-tunnel: w1523 -> [w1527 _]
                  frame Disabled {
                    n650 = Unbundle By Name(w1527) -> ("整组温度不均衡"=w1526:dbl)
                    n651 = call "输入分辨率计算-EV05.vi"("1字节?"=TRUE, "数值"=w1526, "偏移量"=0.0, "分辨率"=1.0) -> ("高字节1"=w1529:dbl)  [unwired: 1 in, 6 out]
                  }
                  frame Enabled {
                  }
                }
                n652 = Build Array(w1525) -> (w1524:i32[])
              }
              frame 5 {
                # "单组电压不均衡"
                n653 = disable-structure shown="启用" {
                  disable-tunnel: [w1541 w1544] -> w1536
                  disable-tunnel: [w1539 w1544] -> w1534
                  disable-tunnel: w1533 -> [w1538 _]
                  frame Disabled {
                    n654 = Unbundle By Name(w1538) -> ("单组电压不均衡"=w1537:dbl)
                    n655 = call "输入分辨率计算-EV05.vi"("1字节?"=FALSE, "数值"=w1537, "偏移量"=0.0, "分辨率"=0.001) -> ("低字节"=w1539:dbl, "高字节1"=w1541:dbl)  [unwired: 1 in, 5 out]
                  }
                  frame Enabled {
                    w1544 = 255 ("高字节1")
                  }
                }
                n656 = Build Array(w1536, w1534) -> (w1535:i32[])
              }
              frame 6 {
                # "整组电压不均衡"
                n657 = disable-structure shown="启用" {
                  disable-tunnel: [w1553 w1556] -> w1548
                  disable-tunnel: [w1551 w1556] -> w1546
                  disable-tunnel: w1545 -> [w1550 _]
                  frame Disabled {
                    n658 = Unbundle By Name(w1550) -> ("整组电压不均衡"=w1549:dbl)
                    n659 = call "输入分辨率计算-EV05.vi"("1字节?"=FALSE, "数值"=w1549, "偏移量"=0.0, "分辨率"=0.001) -> ("低字节"=w1551:dbl, "高字节1"=w1553:dbl)  [unwired: 1 in, 5 out]
                  }
                  frame Enabled {
                    w1556 = 255 ("高字节1")
                  }
                }
                n660 = Build Array(w1548, w1546) -> (w1547:i32[])
              }
              frame 7 {
                # "单体电压过高"
                n661 = disable-structure shown="启用" {
                  disable-tunnel: [w1565 w1568] -> w1560
                  disable-tunnel: [w1563 w1568] -> w1558
                  disable-tunnel: w1557 -> [w1562 _]
                  frame Disabled {
                    n662 = Unbundle By Name(w1562) -> ("单体电压过高"=w1561:dbl)
                    n663 = call "输入分辨率计算-EV05.vi"("1字节?"=FALSE, "数值"=w1561, "偏移量"=0.0, "分辨率"=0.001) -> ("低字节"=w1563:dbl, "高字节1"=w1565:dbl)  [unwired: 1 in, 5 out]
                  }
                  frame Enabled {
                    w1568 = 255 ("高字节1")
                  }
                }
                n664 = Build Array(w1560, w1558) -> (w1559:i32[])
              }
              frame 8 {
                # "单体电压过低"
                n665 = disable-structure shown="启用" {
                  disable-tunnel: [w1577 w1580] -> w1572
                  disable-tunnel: [w1575 w1580] -> w1570
                  disable-tunnel: w1569 -> [w1574 _]
                  frame Disabled {
                    n666 = Unbundle By Name(w1574) -> ("单体电压过低"=w1573:dbl)
                    n667 = call "输入分辨率计算-EV05.vi"("1字节?"=FALSE, "数值"=w1573, "偏移量"=0.0, "分辨率"=0.001) -> ("低字节"=w1575:dbl, "高字节1"=w1577:dbl)  [unwired: 1 in, 5 out]
                  }
                  frame Enabled {
                    w1580 = 255 ("高字节1")
                  }
                }
                n668 = Build Array(w1572, w1570) -> (w1571:i32[])
              }
              frame 9 {
                # "充电电流过高"
                n669 = disable-structure shown="启用" {
                  disable-tunnel: [w1589 w1592] -> w1584
                  disable-tunnel: [w1587 w1592] -> w1582
                  disable-tunnel: w1581 -> [w1586 _]
                  frame Disabled {
                    n670 = Unbundle By Name(w1586) -> ("充电电流过高"=w1585:dbl)
                    n671 = call "输入分辨率计算-EV05.vi"("1字节?"=FALSE, "数值"=w1585, "偏移量"=-3000.0, "分辨率"=0.1) -> ("低字节"=w1587:dbl, "高字节1"=w1589:dbl)  [unwired: 1 in, 5 out]
                  }
                  frame Enabled {
                    w1592 = 255 ("高字节1")
                  }
                }
                n672 = Build Array(w1584, w1582) -> (w1583:i32[])
              }
              frame 10 {
                # "放电电流过高"
                n673 = disable-structure shown="启用" {
                  disable-tunnel: [w1601 w1604] -> w1596
                  disable-tunnel: [w1599 w1604] -> w1594
                  disable-tunnel: w1593 -> [w1598 _]
                  frame Disabled {
                    n674 = Unbundle By Name(w1598) -> ("放电电流过高"=w1597:dbl)
                    n675 = call "输入分辨率计算-EV05.vi"("1字节?"=FALSE, "数值"=w1597, "偏移量"=-3000.0, "分辨率"=0.1) -> ("低字节"=w1599:dbl, "高字节1"=w1601:dbl)  [unwired: 1 in, 5 out]
                  }
                  frame Enabled {
                    w1604 = 255 ("高字节1")
                  }
                }
                n676 = Build Array(w1596, w1594) -> (w1595:i32[])
              }
              frame 11 {
                # "单组温度不均衡"
                n677 = disable-structure shown="启用" {
                  disable-tunnel: [w1611 255 ("高字节1")] -> w1607
                  disable-tunnel: w1605 -> [w1609 _]
                  frame Disabled {
                    n678 = Unbundle By Name(w1609) -> ("单组温度不均衡"=w1608:dbl)
